vi "ActDriveStraightCalcError-ALT Ver 2.vi"(11 "Main Array in":T1={"FIFO Array"=[{"Auto States"=enum."Initilize", "Dist"=4.3, "Radians"=0.0, "MaxSpeed (ft/s)"=1.2, "TimeOut (s)"=10.0, "CMD"="", "ArmSetpoints"=enum."ShoulderRest"}], "Dist (ft)"=0.0, "MaxSpeed (ft/s)"=0.0, "TimeOut (s)"=99.0, "Timer Value"=0, "DriveStraightDistance"=[], "ModuleTravelPosition"=[0.0, 0.0, 0.0, 0.0], "First Time"=FALSE, "Current Step"={"Auto States"=enum."Unknown", "Dist"=4.3, "Radians"=0.0, "MaxSpeed (ft/s)"=1.2, "TimeOut (s)"=10.0, "CMD"="", "ArmSetpoints"=enum."ShoulderRest"}}) -> (1 "Dist Error (Ft)":dbl, 3 "Main Array out":T1={"FIFO Array"=[{"Auto States"=enum."Initilize", "Dist"=4.3, "Radians"=0.0, "MaxSpeed (ft/s)"=1.2, "TimeOut (s)"=10.0, "CMD"="", "ArmSetpoints"=enum."ShoulderRest"}], "Dist (ft)"=0.0, "MaxSpeed (ft/s)"=0.0, "TimeOut (s)"=99.0, "Timer Value"=0, "DriveStraightDistance"=[], "ModuleTravelPosition"=[0.0, 0.0, 0.0, 0.0], "First Time"=FALSE, "Current Step"={"Auto States"=enum."Unknown", "Dist"=4.3, "Radians"=0.0, "MaxSpeed (ft/s)"=1.2, "TimeOut (s)"=10.0, "CMD"="", "ArmSetpoints"=enum."ShoulderRest"}})   [LabVIEW 2023]
uses:
  Auton Main/Auton Main Array.ctl
  Auton Main/State Machine/FIFO Array.ctl
  Auton Main/State Machine/Auot FIFO.ctl
  Auton Main/State Machine/Auot States.ctl
  Shoulder/ShoulderGetSetpointEnum.ctl
  <vilib>/Rock Robotics/Network Tables/NT Write Number.vi
  <vilib>/Rock Robotics/Network Tables/NT Write Numeric Array.vi
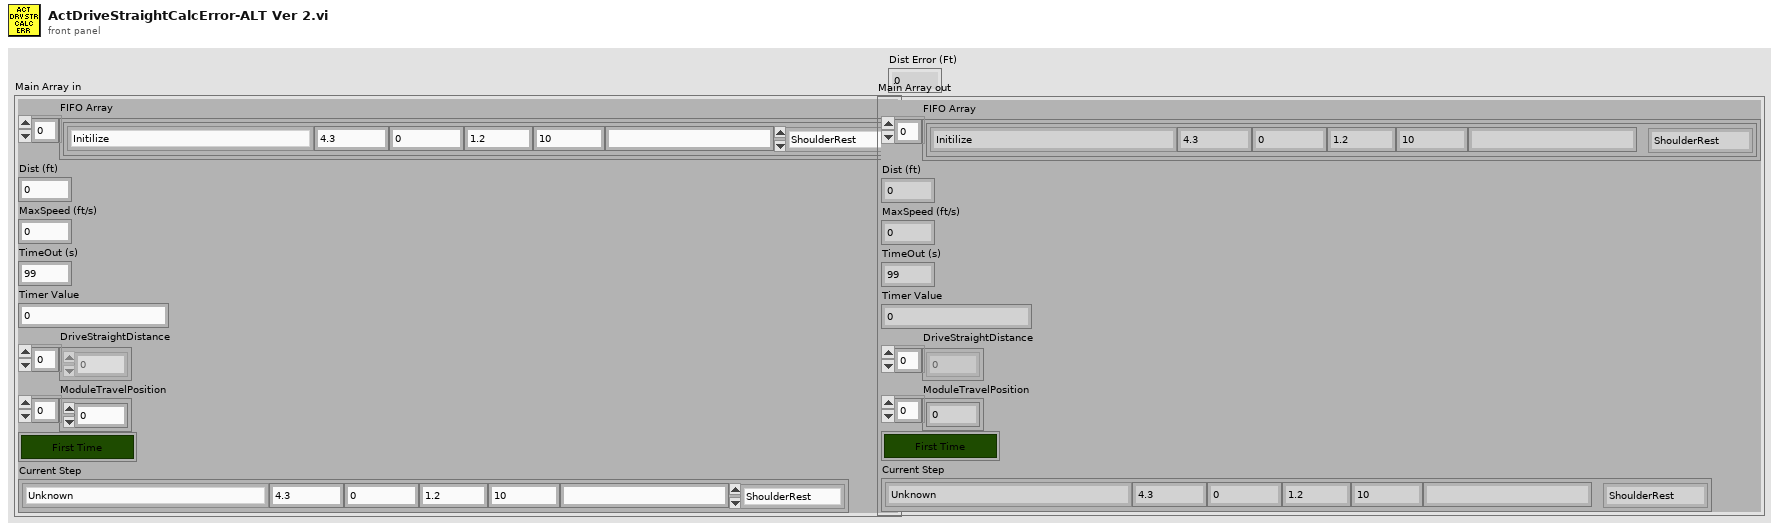
[diagram p1: front panel]
types:
  T1 = typedef "Auton Main Array.ctl" = cluster{"FIFO Array":T2, "Dist (ft)":dbl, "MaxSpeed (ft/s)":dbl, "TimeOut (s)":dbl, "Timer Value":u32, "DriveStraightDistance":dbl[], "ModuleTravelPosition":dbl[], "First Time":bool, "Current Step":T3}
  T2 = typedef "FIFO Array.ctl" = T3[]
  T3 = typedef "Auot FIFO.ctl" = cluster{"Auto States":T4, "Dist":dbl, "Radians":dbl, "MaxSpeed (ft/s)":dbl, "TimeOut (s)":dbl, "CMD":string, "ArmSetpoints":T5}
  T4 = typedef "Auot States.ctl" = enum16{"Unknown", "Initilize", "Intake", "Move Arm", "Drive Straight", "Drive Trajorctory", "Drive Turn", "Send Bool CMD", "Set Target", "Shoot", "Wait", "Exit"}
  T5 = typedef "ShoulderGetSetpointEnum.ctl" = enum16{"Select", "ShoulderRest", "ShoulderSpeaker", "ShoulderAmp"}
  T6 = typedef "Trajectory_Library.lvlib/SWERVE_DRIVE_MODULE_POSITION.ctl" = cluster{"Distance":dbl, "Angle":T7, "P":bool}
  T7 = typedef "Trajectory_Library.lvlib/ROTATION2D.ctl" = cluster{"VALUE":dbl, "COS":dbl, "SIN":dbl}
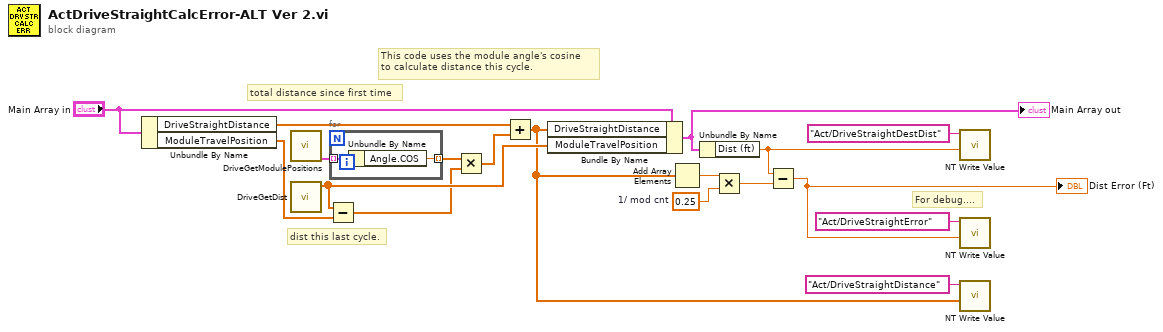
[diagram p0: block diagram]
diagram:
  w18 = 0.25  # 1/ mod cnt
  # "total distance since first time"
  # "dist this last cycle."
  # "For debug...."
  # "This code uses the module angle's cosine\nto calculate distance this cycle."
  n1 = Unbundle By Name("Main Array in") -> ("DriveStraightDistance"=w10:dbl[], "ModuleTravelPosition"=w9:dbl[])
  n2 = call "DriveGetModulePositions.vi"() -> ("Swerve_Drive_Modual_Positions"=w3:T6[])  [unwired: 11 in]
  n3 = call "DriveGetDist.vi"() -> ("ModuleTravelPosition"=w8:dbl[])  [unwired: 11 in]
  n4 = Subtract(x=w8, y=w9) -> (x-y=w5:dbl[])
  n5 = for {
    tunnel: w3 -> [w20] mode=indexing
    tunnel: [w19] -> w6 mode=indexing
    n6 = Unbundle By Name(w20) -> ("Angle.COS"=w19:dbl)
  }
  n7 = Multiply(x=w6, y=w5) -> (x*y=w4:dbl[])
  n8 = Add(x=w10, y=w4) -> (x+y=w7:dbl[])
  n9 = Bundle By Name(cluster="Main Array in", "DriveStraightDistance"=w7, "ModuleTravelPosition"=w8) -> (w1:T1)
  "Main Array out" <- w1
  n10 = Add Array Elements(numeric array=w7) -> (sum=w17:dbl)
  n11 = Unbundle By Name(w1) -> ("Dist (ft)"=w11:dbl)
  n12 = Multiply(x=w17, y=w18) -> (x*y=w16:dbl)
  n13 = Subtract(x=w11, y=w16) -> (x-y=w12:dbl)
  "Dist Error (Ft)" <- w12
  n14 = call-poly <vilib>:"NT Write Value.vi"("value"=w11, "name"="Act/DriveStraightDestDist") -> ()  [unwired: 9 in, 1 out]
  n15 = call-poly <vilib>:"NT Write Value.vi"("value"=w12, "name"="Act/DriveStraightError") -> ()  [unwired: 9 in, 1 out]
  n16 = call-poly <vilib>:"NT Write Value.vi"("value"=w7, "name"="Act/DriveStraightDistance") -> ()  [unwired: 9 in, 1 out]
